vi "Coverage_Error.vi"(8 "error in (no error)":errorcluster caption="entrée d'erreur (pas d'erreur)", 9 "y_score":string[][](array[string]), 10 "y_true":string[][](array[string]), 11 "coverage_error":cluster{"sample_weight":dbl[]}) -> (0 "error out":errorcluster caption="sortie d'erreur", 3 "Score":string)   [LabVIEW 2020]
doc: "Coverage error measure\n\nCompute how far we need to go through the ranked scores to cover all true labels. The best value is equal to the average number of labels in y_true per sample.\n\nTies in y_scores are broken by giving maximal rank that would have been assigned to all tied values.\n\nNote: Our implementation’s score is 1 greater than the one given in Tsoumakas et al., 2010. This extends it to handle the degenerate case in which an instance has 0 true labels.\n\n\n\nParameters : \n\n- y_true : array, shape = [n_samples, n_labels]\nTrue binary labels in binary indicator format.\n\n- y_score : array, shape = [n_samples, n_labels]\nTarget scores, can either be probability estimates of the positive class, confidence values, or non-thresholded measure of decisions (as returned by “decision_function” on some classifiers).\n\n- sample_weight : array-like of shape (n_samples,), default=None\nSample weights.\n\nReturns : \n\n- coverage_error : float"
uses:
  Coverage_Error.lvclass
panel:
  out "Coverage_Error.lvclass":refnum<class "Coverage_Error.lvclass">
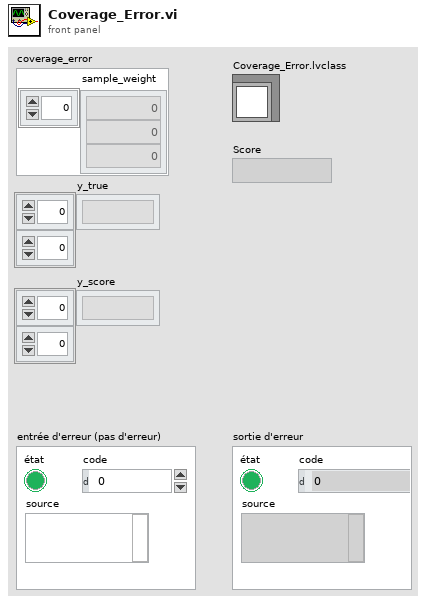
[diagram p1: front panel]
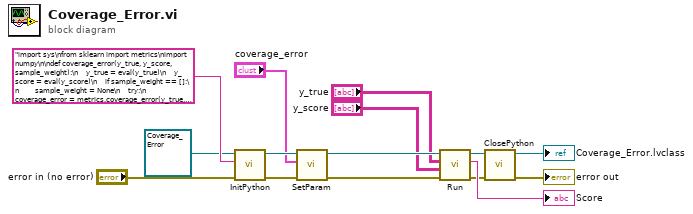
[diagram p0: block diagram]
diagram:
  n1 = call-dynamic "InitPython.vi"("error in (no error)"="error in (no error)", "Python Instruction"="import sys\nfrom sklearn import metrics\nimport numpy\n\ndef coverage_error(y_true, y_score, sample_weight):\n    y_true = eval(y_true)\n    y_score = eval(y_score)\n    if sample_weight == []:\n        sample_weight = None\n    try:\n        coverage_error = metrics.coverage_error(y_true, y_score, sample_weight)\n        coverage_error = coverage_error.tolist()\n        return str(coverage_error)\n    except:\n        erreur = sys.exc_info()\n        typerr = u\"%s\" % (erreur[0])\n        typerr = typerr[typerr.find(\"'\")+1:typerr.rfind(\"'\")]\n        msgerr = u\"%s\" % (erreur[1])\n        message = str('/!\\\\ {0} : {1}'. format(typerr,msgerr))\n        return message", "Scikit-learn en entrée"=refnum<class "Coverage_Error.lvclass"> refnum ("Coverage_Error.lvclass")) -> ("error out"=w11:errorcluster, "Scikit-learn en sortie"=w10:refnum<class "Coverage_Error.lvclass">)  [unwired: 7 in]
  n2 = call-dynamic "SetParam.vi"("error in (no error)"=w11, "coverage_error"="coverage_error", "Coverage_Error.lvclass"=w10) -> ("error out"=w8:errorcluster, "Coverage_Error.lvclass"=w7:refnum<class "Coverage_Error.lvclass">)  [unwired: 7 in]
  n3 = call-dynamic "Run.vi"("error in (no error)"=w8, "y_score"="y_score", "y_true"="y_true", "Coverage_Error.lvclass"=w7) -> ("error out"=w4:errorcluster, "String Data"=→"Score":string, "Coverage_Error.lvclass"=w6:refnum<class "Coverage_Error.lvclass">)  [unwired: 5 in]
  n4 = call-dynamic "ClosePython.vi"("error in (no error)"=w4, "Scikit-learn en entrée"=w6) -> ("error out"=→"error out":errorcluster, "Scikit-learn en sortie"=→"Coverage_Error.lvclass":refnum<class "Coverage_Error.lvclass">)  [unwired: 8 in]
